vi "Synchronize Phase.vi"(8 "error in (no error)":errorcluster, 11 "VISA resource name":refnum<visa-resource-name>) -> (0 "error out":errorcluster, 3 "VISA resource name out":refnum<visa-resource-name>)   [LabVIEW 2009, in "Tektronix AFG 3000 Series.lvlib"]
doc: "Synchronizes the phase of both channels of a (dual-channel) Tektronix AFG 3000 series function generator. <B>Doesn't work yet, for some reason, though it throws no errors.</B>"
uses:
  Tektronix AFG 3000 Series.lvlib
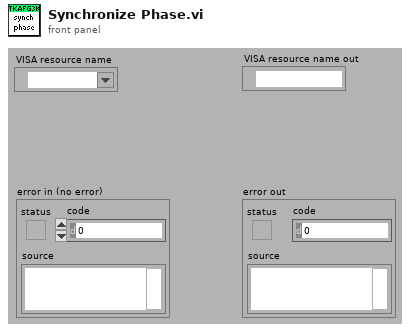
[diagram p1: front panel]
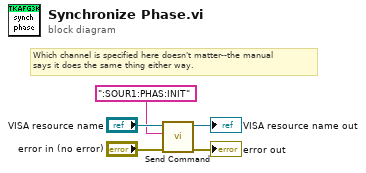
[diagram p0: block diagram]
diagram:
  # "Which channel is specified here doesn't matter--the manual\nsays it does the same thing either way."
  n1 = call "Send Command.vi"("error in (no error)"="error in (no error)", "write buffer"=":SOUR1:PHAS:INIT", "VISA resource name"="VISA resource name") -> ("error out"=→"error out":errorcluster, "VISA resource name out"=→"VISA resource name out":refnum<visa-resource-name>)  [unwired: 7 out]
